vi "Send Command To Host.vi"(6 "Timeout":i32, 7 "Message Priority":T1, 8 "error in (no error)":errorcluster, 10 "Command Message":refnum<class "Command Message Interface.lvclass">, 11 "Mediated Actor in":refnum<class "Mediated Actor.lvclass">) -> (0 "error out":errorcluster, 3 "Mediated Actor out":refnum<class "Mediated Actor.lvclass">)   [LabVIEW 2016, in "Stream Mediator.lvlib" / "Mediated Actor.lvclass"]
doc: "--\nCopyright © 2017 Composed SystemsI All rights reserved.\n\nAuthor: Jon McBee <jon.mcbee@composed.io>\n\nThis library is provided \"AS IS\" ,WITHOUT WARRANTIES OR\nCONDITIONS OF ANY KIND, either express or implied.\n\nComposed Systems -- composed.io\n\nStream 0.0.1.1\nJon McBee - Composed Systems\nCopyright (c) 2017, Composed Systems"
uses:
  <userlib>/Composed Systems/Stream/Mediator/Classes/Mediated Actor/Mediated Actor.lvclass
  C:/Program Files (x86)/National Instruments/LabVIEW 2016/user.lib/Composed Systems/Stream/Actor/Actor Class/Ancestral Actor.lvclass
  <userlib>/Composed Systems/Stream/Mediator/Classes/Message Command Interface/Command Message Interface.lvclass
  C:/Program Files (x86)/National Instruments/LabVIEW 2016/user.lib/Composed Systems/Stream/Mediator/Classes/Message Interface/Message Interface.lvclass
  <userlib>/Composed Systems/Stream/Mediator/Classes/Message Transport Interface/Message Priority.ctl
  <userlib>/Composed Systems/Stream/Actor/Actor Class/Ancestral Actor.lvclass/Ancestral Actor.ctl
  <userlib>/Composed Systems/Stream/Mediator/Classes/Mediated Actor/Mediated Actor.lvclass/Mediated Actor.ctl
  <userlib>/Composed Systems/Stream/Mediator/Classes/Message Command Interface/Command Message Interface.lvclass/Command Message Interface.ctl
  <userlib>/Composed Systems/Stream/Mediator/Classes/Message Transport Queue/Message Transport Queue.lvclass
  <userlib>/Composed Systems/Stream/Actor/Actor Class/Ancestral Actor.lvclass
  <userlib>/Composed Systems/Stream/Mediator/Classes/Message Transport Interface/Message Transport Interface.lvclass
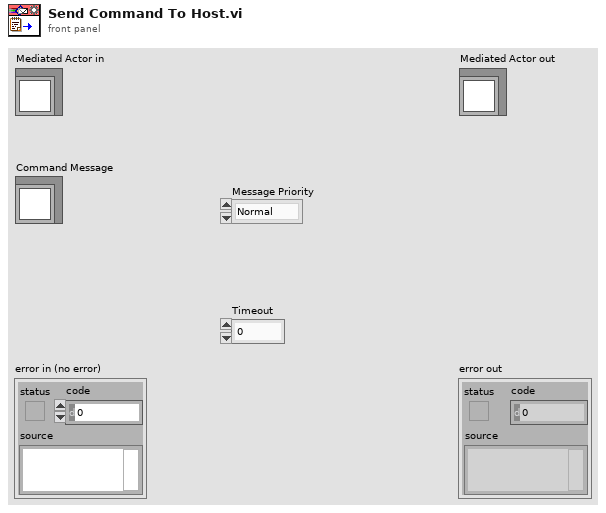
[diagram p1: front panel]
types:
  T1 = typedef "Stream Mediator.lvlib/Message Transport Interface.lvclass/Message Priority.ctl" = enum16{"Normal", "High"}
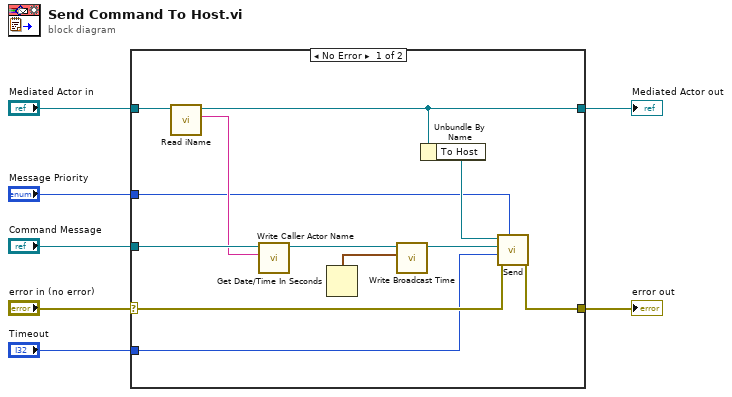
[diagram p0: block diagram]
diagram:
  n1 = case shown="No Error" "error in (no error)" {
    selector: "error in (no error)" -> [w14 w21]
    tunnel: [w13 w21] -> w6
    tunnel: [w10 w20] -> w4
    tunnel: "Mediated Actor in" -> [w19 w20]
    tunnel: "Command Message" -> [w18 _]
    tunnel: "Timeout" -> [w11 _]
    tunnel: "Message Priority" -> [w8 _]
    frame No Error {
      n2 = call <userlib>:"Read iName.vi"("Ancestral Actor in"=w19) -> ("iName"=w16:string, "Ancestral Actor out"=w10:refnum<class "Mediated Actor.lvclass">)  [unwired: 8 in, 1 out]
      n3 = call <userlib>:"Write Caller Actor Name.vi"("Caller Actor Name"=w16, "Command Message Interface in"=w18) -> ("Command Message Interface out"=w17:refnum<class "Command Message Interface.lvclass">)  [unwired: 9 in]
      n4 = Get Date/Time In Seconds() -> (seconds since 1Jan1904=w15:timestamp)
      n5 = call <userlib>:"Write Broadcast Time.vi"("Broadcast Time"=w15, "Command Message Interface in"=w17) -> ("Command Message Interface out"=w12:refnum<class "Command Message Interface.lvclass">)  [unwired: 9 in]
      n6 = Unbundle By Name(w10) -> ("To Host"=w9:refnum<class "Message Transport Queue.lvclass">)
      n7 = call-dynamic "Send.vi"("Message Priority"=w8, "error in (no error)"=w14, "Timeout"=w11, "Message"=w12, "Message Transport Queue in"=w9) -> ("error out"=w13:errorcluster)  [unwired: 4 in, 2 out]
    }
    frame Error {
    }
  }
  "error out" <- w6
  "Mediated Actor out" <- w4
